vi "Test TestSuite Segment Contain Execution Time Field.vi"(8 "error in (no error)":errorcluster, 11 "XML Report Test in":refnum<class "XML Report Test.lvclass">) -> (0 "error out":errorcluster, 3 "XML Report Test out":refnum<class "XML Report Test.lvclass">)   [LabVIEW 2020, in "XML Report Test.lvclass"]
uses:
  XML Report Test.lvclass
  XML Report Test.lvclass/XML Report Test.ctl
  source/Plugins/XML Report/XML Report.lvclass
panel:
  out "Report Content":string
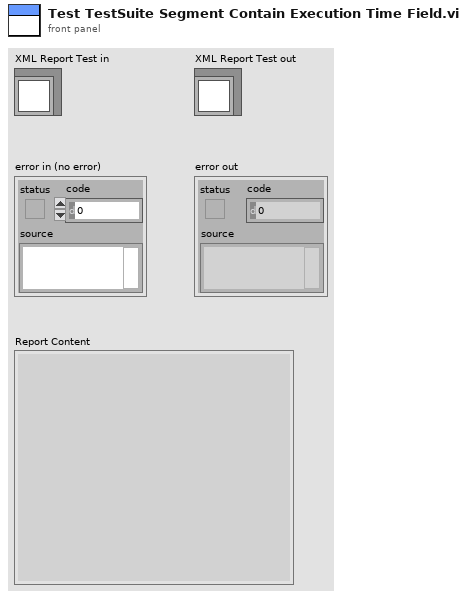
[diagram p1: front panel]
types:
  T1 = typedef "Result.lvlib/Result.ctl" = cluster{"Name":string, "Description":string, "Status":T2, "Result Type":T3, "Execution Time":dbl, "Data":cluster{"Expected":variant, "Actual":variant, "Delta":variant}}
  T2 = typedef "Result.lvlib/Status.ctl" = enum16{"", "Passed", "Failed", "Error", "Skipped", "Setup Error", "Broken", "Teardown Error"}
  T3 = typedef "Result.lvlib/Type.ctl" = enum16{"Test Case", "Test Suite", "Test Run", "Pass", "Fail", "Skip", "Pass if", "Fail if", "Pass if Error", "Fail if Error", "Pass if Equal", "Fail if Equal"}
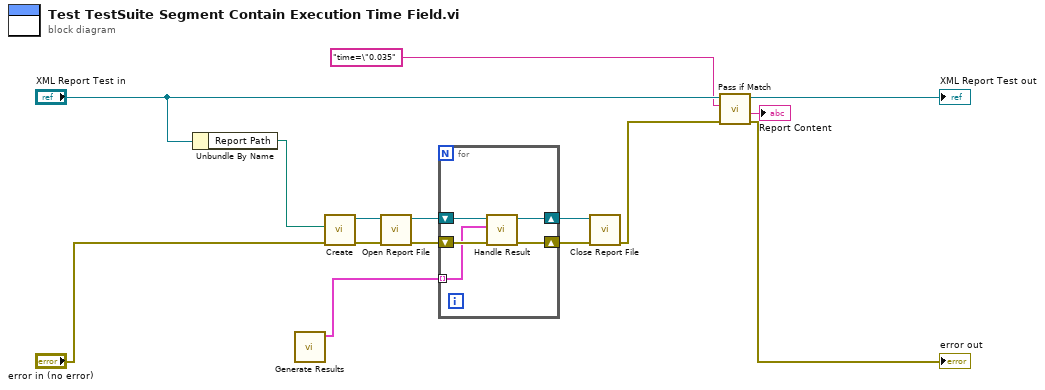
[diagram p0: block diagram]
diagram:
  n1 = Unbundle By Name("XML Report Test in") -> ("Report Path"=w1:path)
  n2 = call "Generate Results.vi"() -> ("Data"=w5:T1[])  [unwired: 10 in, 1 out]
  n3 = call "Create.vi"("error in (no error)"="error in (no error)", "Report Path"=w1) -> ("error out"=w3:errorcluster, "XML Report"=w2:refnum<class "XML Report.lvclass">)  [unwired: 8 in]
  n4 = call-dynamic "Open Report File.vi"("error in (no error)"=w3, "XML Report In"=w2) -> ("error out"=w15:errorcluster, "XML Report Out"=w7:refnum<class "XML Report.lvclass">)  [unwired: 8 in]
  n5 = for {
    shift-right: [w19] -> w8
    shift-left: w15 -> [w20]
    shift-right: [w17] -> w6
    shift-left: w7 -> [w18]
    tunnel: w5 -> [w16] mode=indexing
    n6 = call-dynamic "Handle Result.vi"("error in (no error)"=w20, "Result"=w16, "XML Report In"=w18) -> ("error out"=w19:errorcluster, "XML Report Out"=w17:refnum<class "XML Report.lvclass">)  [unwired: 7 in]
  }
  n7 = call-dynamic "Close Report File.vi"("error in (no error)"=w8, "XML Report In"=w6) -> ("error out"=w11:errorcluster)  [unwired: 8 in, 1 out]
  n8 = call "Pass if Match.vi"("error in (no error)"=w11, "regular expression"="time=\"0.035", "XML Report Test in"="XML Report Test in") -> ("error out"=→"error out":errorcluster, "Report Content"=→"Report Content":string, "XML Report Test out"=→"XML Report Test out":refnum<class "XML Report Test.lvclass">)  [unwired: 6 in]
